vi "Temporizador.vi"() -> ()   [LabVIEW 2020]
panel:
  in  "stop":bool
  out "Elapsed Time (s)":dbl
  out "Time has Elapsed":bool
  in  "Auto Reset":bool=TRUE
  in  "Reset":bool
  in  "Time Target (s)":dbl=1.0
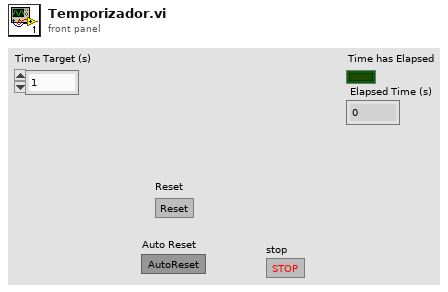
[diagram p1: front panel]
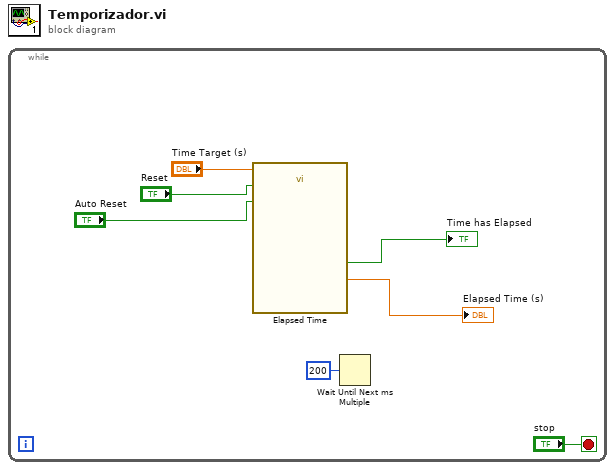
[diagram p0: block diagram]
diagram:
  n1 = while {
    stop <- "stop" stop-if-true
    n2 = call "Elapsed Time"("Time Target (s)"="Time Target (s)", "Reset"="Reset", "Auto Reset"="Auto Reset") -> ("Elapsed Time (s)"=→"Elapsed Time (s)":dbl, "Time has Elapsed"=→"Time has Elapsed":bool)  [unwired: 9 in, 6 out]
    n3 = Wait Until Next ms Multiple(millisecond multiple=u32 200) -> ()  [unwired: 1 out]
  }
